vi "STAT2 decode Digital data from Controller.vi"(10 "Controller Data":T2 {"High G monitoring" format="%02x"; "NA" format="%02x"; "GPIO values" format="%02x"; "Relay status" format="%02x"; "sys register" format="%04x"}) -> (2 "Digital Data Out":T1[](array[typedef]))   [LabVIEW 2011]
uses:
  LEINmaster/Nodes/Controller local stat2.ctl
  Measurments Handling/Status Digitalish.ctl
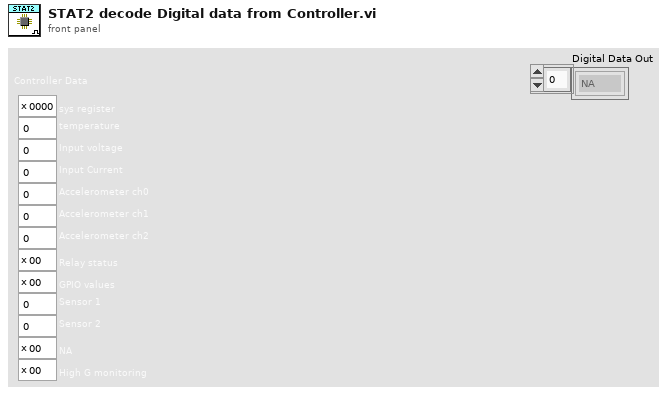
[diagram p1: front panel]
types:
  T1 = typedef "Status Digitalish.ctl" = enum16{"NA", "False", "True"}
  T2 = typedef "Controller local stat2.ctl" = cluster{"sys register":u16, "temperature":u16, "Input voltage":u16, "Input Current":u16, "Accelerometer ch0":u16, "Accelerometer ch1":u16, "Accelerometer ch2":u16, "Relay status":u8, "GPIO values":u8, "Sensor 1":i32, "Sensor 2":i32, "NA":u8, "High G monitoring":u8}
  T3 = typedef "Stat2 system error.ctl" = cluster{"Error":bool, "Has had error":bool, "Com. issue":bool}
  T4 = typedef "Stat2 system task info.ctl" = cluster{"Task":bool, "Task error":bool, "Task cnt.":u8, "Job 0":bool, "User":bool}
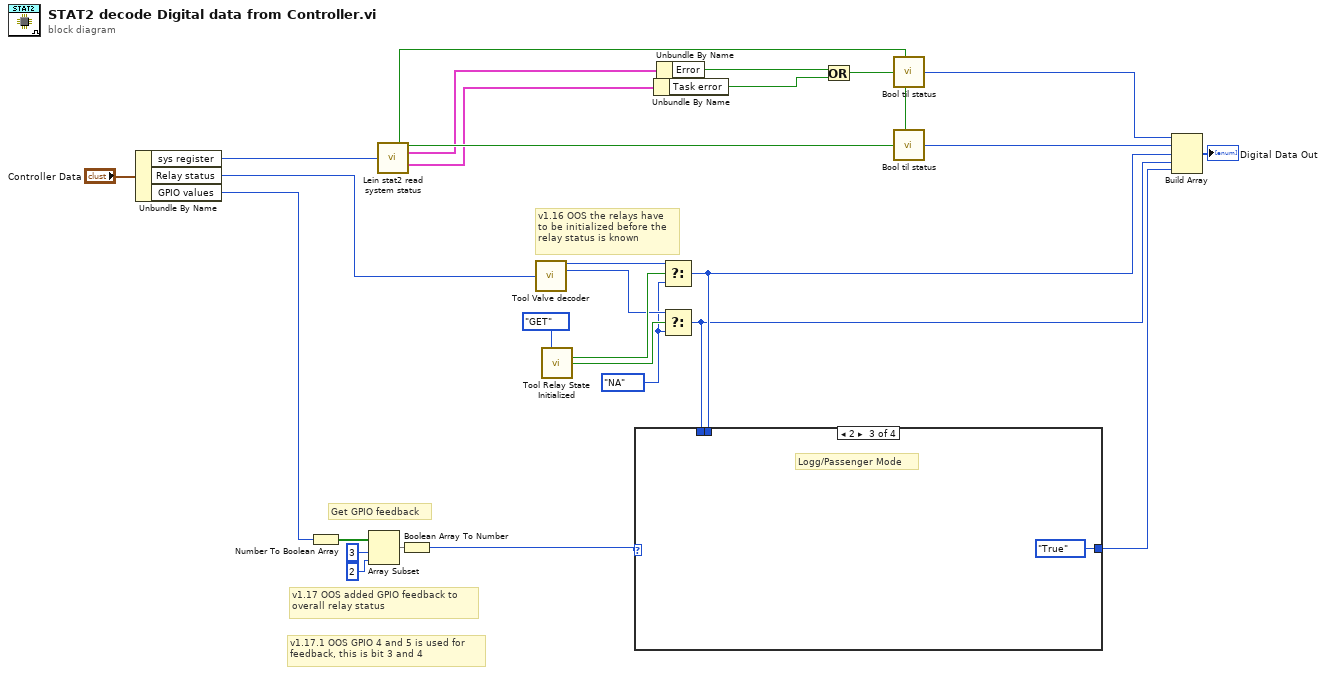
[diagram p0: block diagram]
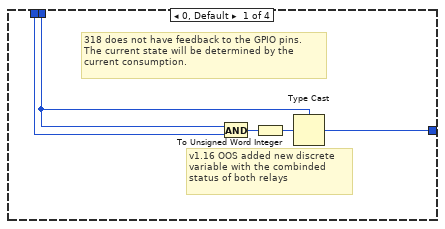
[diagram p2: hidden frame]
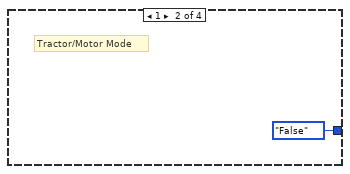
[diagram p3: hidden frame]
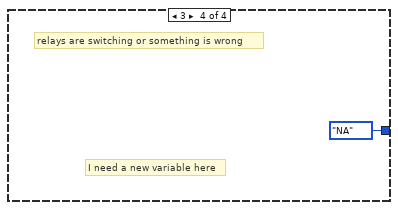
[diagram p4: hidden frame]
diagram:
  w2 = Status_Digitalish."NA" ("f")
  # "v1.17.1 OOS GPIO 4 and 5 is used for \nfeedback, this is bit 3 and 4"
  # "v1.17 OOS added GPIO feedback to\noverall relay status"
  # "v1.16 OOS the relays have \nto be initialized before the \nrelay status is known"
  # "Get GPIO feedback"
  n1 = Unbundle By Name("Controller Data") -> ("sys register"=w27:u16, "Relay status"=w19:u8, "GPIO values"=w12:u8)
  n2 = Number To Boolean Array(number=w12) -> (Boolean array=w9:bool[])
  n3 = Array Subset(array=w9, index=3, length=2) -> (w11:bool[])
  n4 = call "Lein stat2 read system status.vi"("sys register"=w27) -> ("Force NA"=w20:bool, "Stopped"=w26:bool, "Error"=w22:T3, "Task"=w21:T4)  [unwired: 7 in, 4 out]
  n5 = Boolean Array To Number(Boolean array=w11) -> (number=w1:u32)
  n6 = call "Tool Valve decoder.vi"("Valve Relay code"=w19) -> ("Valve LSB(0)"=w4:T1, "Valve 1"=w3:T1)  [unwired: 10 in, 3 out]
  n7 = call "Tool Relay State Initialized.vi"("Action(GET)"=enum16{"GET", "SET"}."GET") -> ("Relay 1 Initialized out"=w6:bool, "Relay 2 Initialized out"=w5:bool)  [unwired: 12 in, 1 out]
  n8 = Unbundle By Name(w21) -> ("Task error"=w25:bool)
  n9 = Unbundle By Name(w22) -> ("Error"=w23:bool)
  n10 = Select(t=w4, s=w6, f=w2) -> (s? t:f=w14:T1)
  n11 = Select(t=w3, s=w5, f=w2) -> (s? t:f=w13:T1)
  n12 = case shown="2" w1 {
    tunnel: [w33 Status_Digitalish."False" ("f") Status_Digitalish."True" ("f") Status_Digitalish."NA" ("f")] -> w15
    tunnel: w14 -> [w32 _ _ _]
    tunnel: w13 -> [w31 _ _ _]
    frame 0, Default {
      # "318 does not have feedback to the GPIO pins. \nThe current state will be determined by the \ncurrent consumption."
      # "v1.16 OOS added new discrete \nvariable with the combinded \nstatus of both relays"
      n13 = And(x=w32, y=w31) -> (x .and. y?=w29:i32)
      n14 = To Unsigned Word Integer(number=w29) -> (unsigned 16bit integer=w30:u16)
      n15 = Type Cast(type=w32, x=w30) -> (*(type *) &x=w33:T1)
    }
    frame 1 {
      # "Tractor/Motor Mode"
    }
    frame 2 {
      # "Logg/Passenger Mode"
    }
    frame 3 {
      # "I need a new variable here"
      # "relays are switching or something is wrong"
    }
  }
  n16 = Or(x=w23, y=w25) -> (x .or. y?=w24:bool)
  n17 = call "Bool til status.vi"("Force NA(F)"=w20, "Boolean"=w24) -> ("Status"=w18:T1)  [unwired: 7 in]
  n18 = call "Bool til status.vi"("Force NA(F)"=w20, "Boolean"=w26) -> ("Status"=w17:T1)  [unwired: 7 in]
  n19 = Build Array(w18, w17, w14, w13, w15) -> (→"Digital Data Out":T1[])
